vi "LabvolutionSubmoduleCheck_GitReset.vi"(8 "error in (no error)":errorcluster, 11 "Working Dir in":path) -> (0 "error out":errorcluster, 2 "Command OK":bool, 3 "Working Dir out":path)   [LabVIEW 2018]
uses:
  callback-system-exec/callback-system-exec/callback-system-exec.lvlib
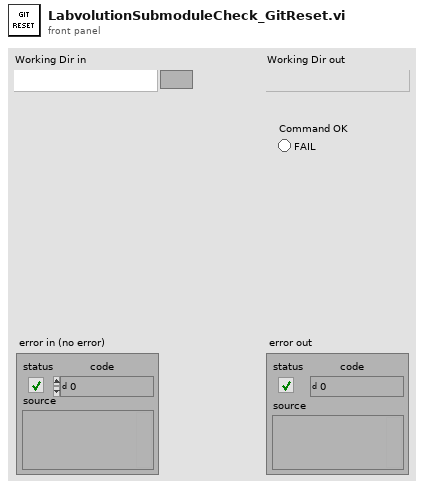
[diagram p1: front panel]
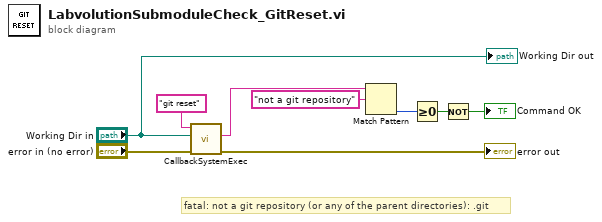
[diagram p0: block diagram]
diagram:
  # "fatal: not a git repository (or any of the parent directories): .git"
  n1 = call "CallbackSystemExec.vi"("error in (no error)"="error in (no error)", "Working directory"="Working Dir in", "Command"="git reset") -> ("error out"=→"error out":errorcluster, "Standard Error"=w1:string)  [unwired: 6 in, 1 out]
  n2 = Match Pattern(string=w1, regular expression="not a git repository") -> (offset past match=w8:i32)  [unwired: 1 in, 3 out]
  n3 = Greater Or Equal To 0?(x=w8) -> (x >= 0?=w7:bool)
  n4 = Not(x=w7) -> (.not. x?=→"Command OK":bool)
  "Working Dir out" <- "Working Dir in"
